vi "1st CMD Operations.vi"(8 "error in (no error)":errorcluster, 10 "Message In":refnum<class "Message.lvclass">, 11 "UI Console in":refnum<class "UI Console.lvclass">) -> (0 "error out":errorcluster, 2 "Stop":bool, 3 "UI Console out":refnum<class "UI Console.lvclass">)   [LabVIEW 2024, in "UI Console.lvclass"]
uses:
  UI Console.lvclass
  Ancestor Class/Message/Message.lvclass
  UI Console MSG/UI Console MSG.lvclass
  UI Console MSG/UI Console MSG.lvclass/UI Console MSG.ctl
  UI Console MSG/Public Data/Read UI Console 1st CMD.vi
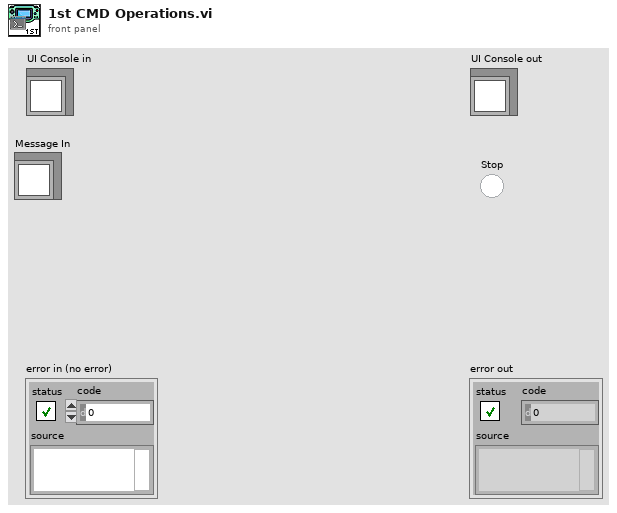
[diagram p1: front panel]
types:
  T1 = typedef "UI Console 1st CMD.ctl" = enum16{"None", "UI Manipulation", "UI Operation", "UI Stop"}
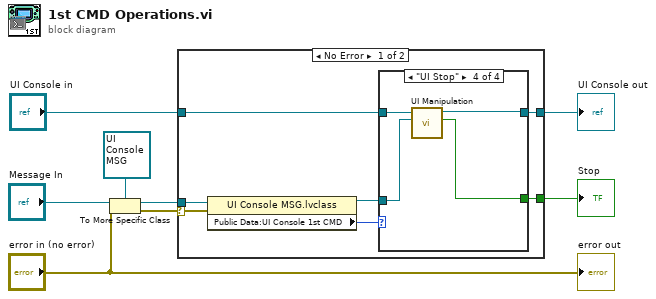
[diagram p0: block diagram]
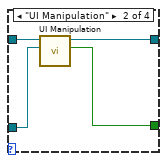
[diagram p3: hidden frame]
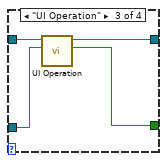
[diagram p4: hidden frame]
diagram:
  n1 = To More Specific Class(target class=refnum<class "UI Console MSG.lvclass"> refnum ("UI Console MSG.lvclass"), reference="Message In", error in="error in (no error)") -> (specific class reference=w2:refnum<class "UI Console MSG.lvclass">, error out=w6:errorcluster)
  n2 = case shown="No Error" w6 {
    selector: w6 -> [w15 _]
    tunnel: "UI Console in" -> [w12 w29]
    tunnel: [w11 w29] -> w4
    tunnel: w2 -> [w14 _]
    tunnel: [w9 _] -> w1
    frame No Error {
      n3 = property class="UI Console MSG.lvclass"(reference=w14, error in=w15) -> (reference out=w10:refnum<class "UI Console MSG.lvclass">, "Public Data:UI Console 1st CMD"=w13:T1)  [unwired: 1 out]
      n4 = case shown="\"UI Stop\"" w13 {
        tunnel: w12 -> [w16 w20 w24 w28]
        tunnel: [w16 w19 w22 w26] -> w11
        tunnel: w10 -> [_ w18 w23 w27]
        tunnel: [_ w17 w21 w25] -> w9
        frame "None", Default {
        }
        frame "UI Manipulation" {
          n5 = call-dynamic "UI Manipulation.vi"("UI Console MSG In"=w18, "UI Console in"=w20) -> ("Stop"=w17:bool, "UI Console out"=w19:refnum<class "UI Console.lvclass">)  [unwired: 7 in, 1 out]
        }
        frame "UI Operation" {
          n6 = call-dynamic "UI Operation.vi"("UI Console MSG In"=w23, "UI Console in"=w24) -> ("Stop"=w21:bool, "UI Console out"=w22:refnum<class "UI Console.lvclass">)  [unwired: 7 in, 1 out]
        }
        frame "UI Stop" {
          n7 = call-dynamic "UI Manipulation.vi"("UI Console MSG In"=w27, "UI Console in"=w28) -> ("Stop"=w25:bool, "UI Console out"=w26:refnum<class "UI Console.lvclass">)  [unwired: 7 in, 1 out]
        }
      }
    }
    frame Error {
    }
  }
  "UI Console out" <- w4
  "Stop" <- w1
  "error out" <- "error in (no error)"
